vi "Jenn_WiFiNode.vi"() -> ()   [LabVIEW 2016]
uses:
  VIs/uPythonX/uPythonX.xctl
panel:
  in  "Main":T1(xcontrol)={"VISA Refnum in"="ASRL44::INSTR", "All Code"="#####\n# Browser Programmable Feather\n# Based on code from ShrimpingIt/cockle https://github.com/ShrimpingIt/cockle/tree/master/replserver\n#\n# Jennifer Cross\n# December 2018\n####\nimport network\nimport os\nimport gc\nimport ubinascii\nimport ure\nimport webrepl\n\ntry:\n     import usocket as socket\nexcept:\n     import socket\n     \ngc.collect()\n\nwl_ap = network.WLAN(1)\nwl_ap.config(essid='PYBD')          # set AP SSID\nwl_ap.config(password='pybd0123')   # set AP password\nwl_ap.config(channel=6)             # set AP channel\nwl_ap.active(1)                     # enable the AP\n\nwl_ap.status('stations')    # get a list of connection stations\n\nmac = ubinascii.hexlify(network.WLAN().config('mac'),':').decode()\nprint(\"This device has MAC address: \" + mac)\n\nssidshort = mac[-8:-6]+mac[-5:-3]+mac[-2:]\n\nprint(\"This device is broadcasting the SSID: MicroPython-\" + ssidshort)\nprint(\"This connect to MicroPython\" + ssidshort + \" with password micropythoN\")\n\nwpassword = 'jumbo'\nwebrepl.start(password=wpassword)\nprint(\"Creating WebREPL instance. WebREPL password: \" + wpassword)\n     \nreplpath = \"webrepl-inlined.html.gz\"\n\ns = socket.socket()\nai = socket.getaddrinfo(\"0.0.0.0\", 80)\naddr = ai[0][-1]\n\ns.setsockopt(socket.SOL_SOCKET, socket.SO_REUSEADDR, 1)\ns.bind(addr)\ns.listen(5)\n\nprint(\"Running a local WebREPL server, please connect to 192.168.4.1\")\n\ndef accept_handler(sock):\n     res = sock.accept()\n     print(\"Handling\")\n     client_s = res[0]\n     string_request = client_s.recv(2048).decode('utf-8')\n     #print(\"Request:\" + string_request)\n     try:\n          request_line = string_request.split(\"\\r\\n\")[0]    # only consider first line\n          request_line = request_line.split()     # separate by whitespace \n          (request_method, path, request_version) = request_line\n          header = ''\n          content = ''\n          if request_method == \"GET\" and \"favicon\" not in path:\n               #print(\"GET \"+ path)\n               header += 'HTTP/1.1 200 OK\\r\\n'\n               header += 'Content-Type: text/html; charset=UTF-8\\r\\n'\n               header += 'Content-Encoding: gzip\\r\\n'\n\n               replsize = os.stat(replpath)[6]\n               header += 'Content-Length: ' + str(replsize) + '\\r\\n'\n               header += '\\r\\n'\n\n               client_s.send(header)\n               #print(\"Sent \"+ header)\n               \n               with open(replpath, 'r') as f:\n                    chunkCount = 0\n                    while True:\n                         # TODO CH use buffer and readinto\n                         chunk = f.read(1024)\n                         if chunk != '':\n                              client_s.write(chunk)\n                              #print(\"Sent chunk \" + str(chunkCount) + \":\" + str(len(chunk)))\n                              chunkCount = chunkCount + 1\n                         else:\n                              #print(\"Last chunk sent\")\n                              break                                   \n     except Exception as e:\n          print(\"Exception\", e)\n     finally:\n          client_s.close()\n\ns.setsockopt(socket.SOL_SOCKET, 20, accept_handler)\n\ngc.collect()\n\n# wl_ap.active(0)             # shut down the AP\n"}
  # "This will not run in rawREPL - need to save it as main.oy"
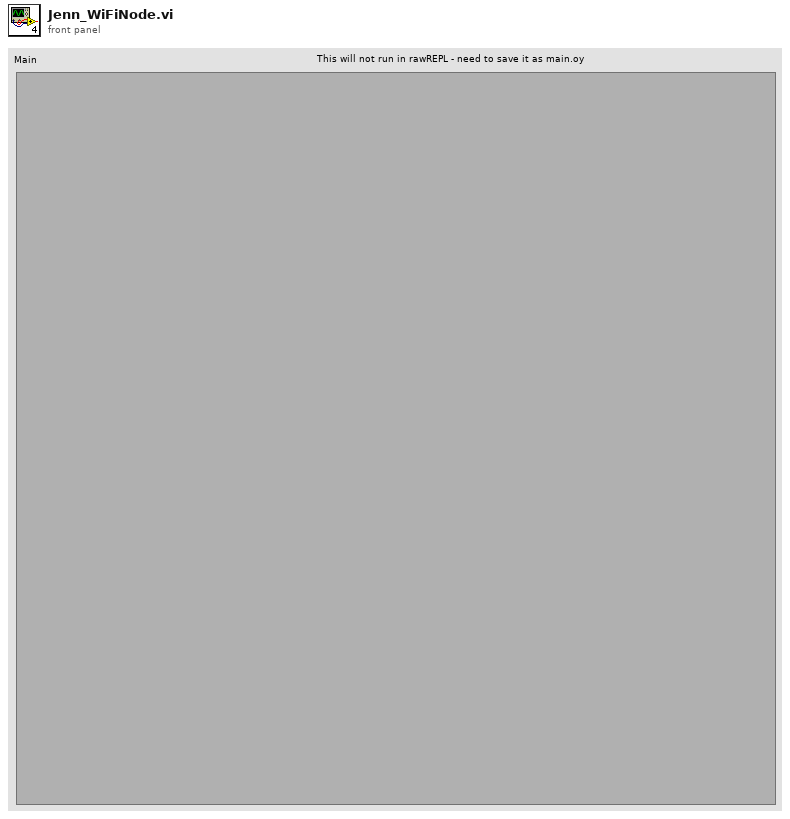
[diagram p1: front panel]
types:
  T1 = cluster{"VISA Refnum in":refnum<visa-resource-name>, "All Code":string}
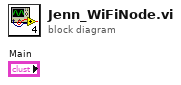
[diagram p0: block diagram]
diagram:
